vi "data-time-expand-by-fitting.vi"(1 "Num of Samples":dbl, 2 "fitting\nmethod":i32(ring)=1 items=["nearest", "linear", "spline", "cubic Hermite", "Lagrange"], 3 "data in":dbl[][](array[numeric])) -> (0 "data out":dbl[][](array[numeric]))   [LabVIEW 2016]
uses:
  <vilib>/Analysis/1siggen.llb/Ramp Pattern by Samples.vi
  <vilib>/Analysis/NI_AALBase.lvlib
  <vilib>/gmath/NI_Gmath.lvlib
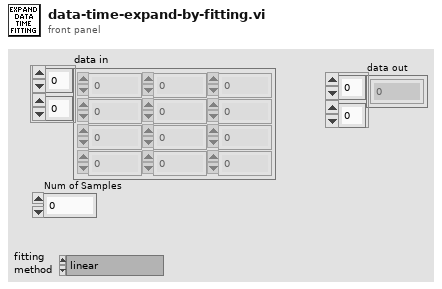
[diagram p1: front panel]
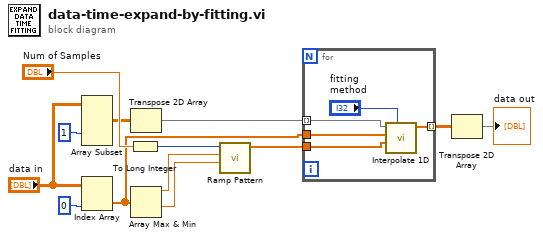
[diagram p0: block diagram]
diagram:
  n1 = Array Subset(array="data in", index (col)=1 ("index")) -> (w5:dbl[][])  [unwired: 3 in]
  n2 = Index Array(array="data in", index (col)=0 ("disabled index (col)")) -> (element=w4:dbl[])  [unwired: 1 in]
  n3 = To Long Integer(number="Num of Samples") -> (32bit integer=w7:i32)
  n4 = Transpose 2D Array(2D array=w5) -> (transposed array=w1:dbl[][])
  n5 = Array Max & Min(array=w4) -> (max value=w8:dbl, min value=w9:dbl)  [unwired: 2 out]
  n6 = call-poly <vilib>:"Ramp Pattern.vi"("start"=w9, "end"=w8, "samples"=w7) -> ("Ramp Pattern"=w3:dbl[])  [unwired: 7 in, 1 out]
  n7 = for {
    tunnel: w1 -> [w18] mode=indexing
    tunnel: w4 -> [w17]
    tunnel: w3 -> [w16]
    tunnel: [w15] -> w2 mode=indexing
    n8 = call <vilib>:"Interpolate 1D.vi"("method"="fitting\nmethod", "xi"=w16, "X"=w17, "Y"=w18) -> ("yi"=w15:dbl[])  [unwired: 5 in, 2 out]
  }
  n9 = Transpose 2D Array(2D array=w2) -> (transposed array=→"data out":dbl[][])
